vi "doubleclick action.vi"(6 "user event":T1, 7 "Row":i32, 8 "error in":errorcluster, 9 "channel list":refnum<vi>, 10 "engine configuration in":refnum<class "engine configuration.lvclass">, 11 "UI Reference configuration in":refnum<class "io configuration.lvclass">) -> (0 "error out":errorcluster, 2 "engine configuration out":refnum<class "engine configuration.lvclass">, 3 "UI Reference configuration out":refnum<class "io configuration.lvclass">)   [LabVIEW 2014, in "io editor node.lvclass"]
uses:
  io editor node.lvclass
  <vilib>/NI/Module Execution Interface/Engine Configuration/engine configuration.lvclass
  <vilib>/NI/Configuration Framework/Controls/EventCluster.ctl
  <vilib>/NI/Configuration Framework/NISE_CEF_TreeControl.lvlib
  <vilib>/NI/Configuration Framework/Node/UserEventRef.ctl
  <vilib>/NI/Configuration Framework/Node/NISE_CEF_Node.lvclass
  configuration/io configuration.lvclass
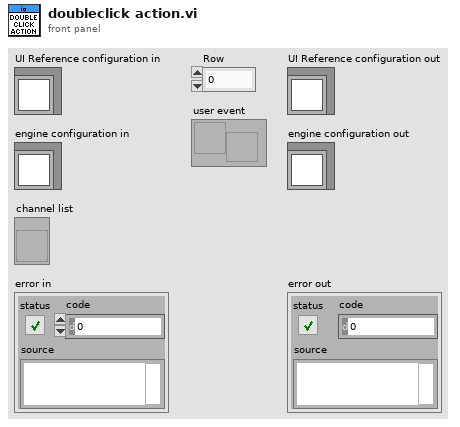
[diagram p1: front panel]
types:
  T1 = typedef "NISE_CEF_Node.lvclass/UserEventRef.ctl" = refnum<user-event>
  T2 = typedef "io editor node.lvclass/table line.ctl" = cluster{"channel":refnum<class "TBM channel.lvclass">, "tag name":string}
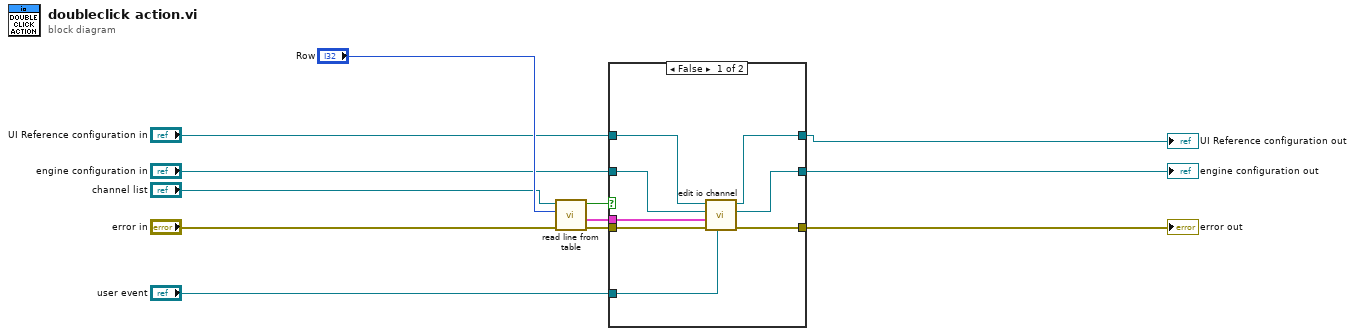
[diagram p0: block diagram]
diagram:
  n1 = call "read line from table.vi"("error in"="error in", "line number"="Row", "channels table"="channel list") -> ("error out"=w3:errorcluster, "line"=w4:T2, "empty channel?"=w10:bool)  [unwired: 5 in, 1 out]
  n2 = case shown="False" w10 {
    tunnel: [w20 w21] -> w2
    tunnel: w3 -> [w19 w21]
    tunnel: w4 -> [w18 _]
    tunnel: "engine configuration in" -> [w17 w22]
    tunnel: "UI Reference configuration in" -> [w16 w23]
    tunnel: [w15 w23] -> w12
    tunnel: [w14 w22] -> w11
    tunnel: "user event" -> [w13 _]
    frame False {
      n3 = call "edit io channel.vi"("user event"=w13, "error in"=w19, "line"=w18, "engine configuration in"=w17, "tag bus configurable plugin module configuration in"=w16) -> ("error out"=w20:errorcluster, "engine configuration"=w14:refnum<class "engine configuration.lvclass">, "tag bus configurable plugin module configuration out"=w15:refnum<class "io configuration.lvclass">)  [unwired: 4 in]
    }
    frame True {
    }
  }
  "UI Reference configuration out" <- w12
  "engine configuration out" <- w11
  "error out" <- w2
